vi "Main_Receiver_Localtest.vi"(7 "Tx IQ Sampling\nRate [s/sec]":dbl, 8 "Bitstream Queue Name":string, 9 "Packet Parameters in":T2={"Length of sync sequence (50)"=50, "Number of message bits"=128, "Number of guardbits"=40, "Sync PN sequence order (31)"=31, "Number of header bits"=16, "Packet Pad [samples]"=0}, 10 "QPSK System Parameters":T4={"Samples per Symbol"=8, "symbol map"=[], "Differential PSK"=enum."disable", "PSK type"=0, "M-PSK"=4} {"PSK type" items=["normal", "shifted", "offset"]; "symbol map" format="%.3f"}, 11 "Waveform Queue Name":string) -> ()   [LabVIEW 2014]
uses:
  <instrlib>/niUSRP/niUSRP Fetch Rx Data (CDB Cluster).vi
  <vilib>/addons/Modulation/Digital/General/MT Format Eye Diagram (complex).vi
  <vilib>/addons/Modulation/niDMT.lvlib
panel:
  out "Waveform Graph":dbl[](graph)
  out "Eye Diagram":cluster{"t0":dbl, "dt":dbl, "Y":dbl[]}[](graph)
  out "Sync start":dbl
  out "Max Xcorr Value":dbl
  in  "output cluster":T1
  out "Frames decoded":i32
  out "Max Xcorr Index":i32
  in  "stop":bool
  out "error out":errorcluster
  in  "error in (no error)":errorcluster
  in  "filter parameters":T3={"Alpha"=0.5, "Filter Length"=6, "TX Filter"=enum."Root Raised Cos"} {"Alpha" format="%.2f"}
  in  "USRP IP Address 2":refnum<k15>="192.168.10.1"
  out "Actual Rx Parameters  2":T5={"Rx IQ Sampling\nRate [s/sec]"=200000.0, "Rx\nFrequency [Hz]"=915000000.0, "Rx Gain [dB]"=20.0, "Rx Antenna"="RX1"} {"Rx Gain [dB]" format="%#.6p"; "Rx\nFrequency [Hz]" format="%#.6p"; "Rx IQ Sampling\nRate [s/sec]" format="%#.6p"}
  in  "Rx Parameters 2":T5={"Rx IQ Sampling\nRate [s/sec]"=400000.0, "Rx\nFrequency [Hz]"=5795000000.0, "Rx Gain [dB]"=20.0, "Rx Antenna"="RX1"} {"Rx Gain [dB]" format="%#.6p"; "Rx\nFrequency [Hz]" format="%#.6p"; "Rx IQ Sampling\nRate [s/sec]" format="%#.6p"}
  in  "Acquisition Duration [sec] 2":dbl=0.04 format="%#.6p"
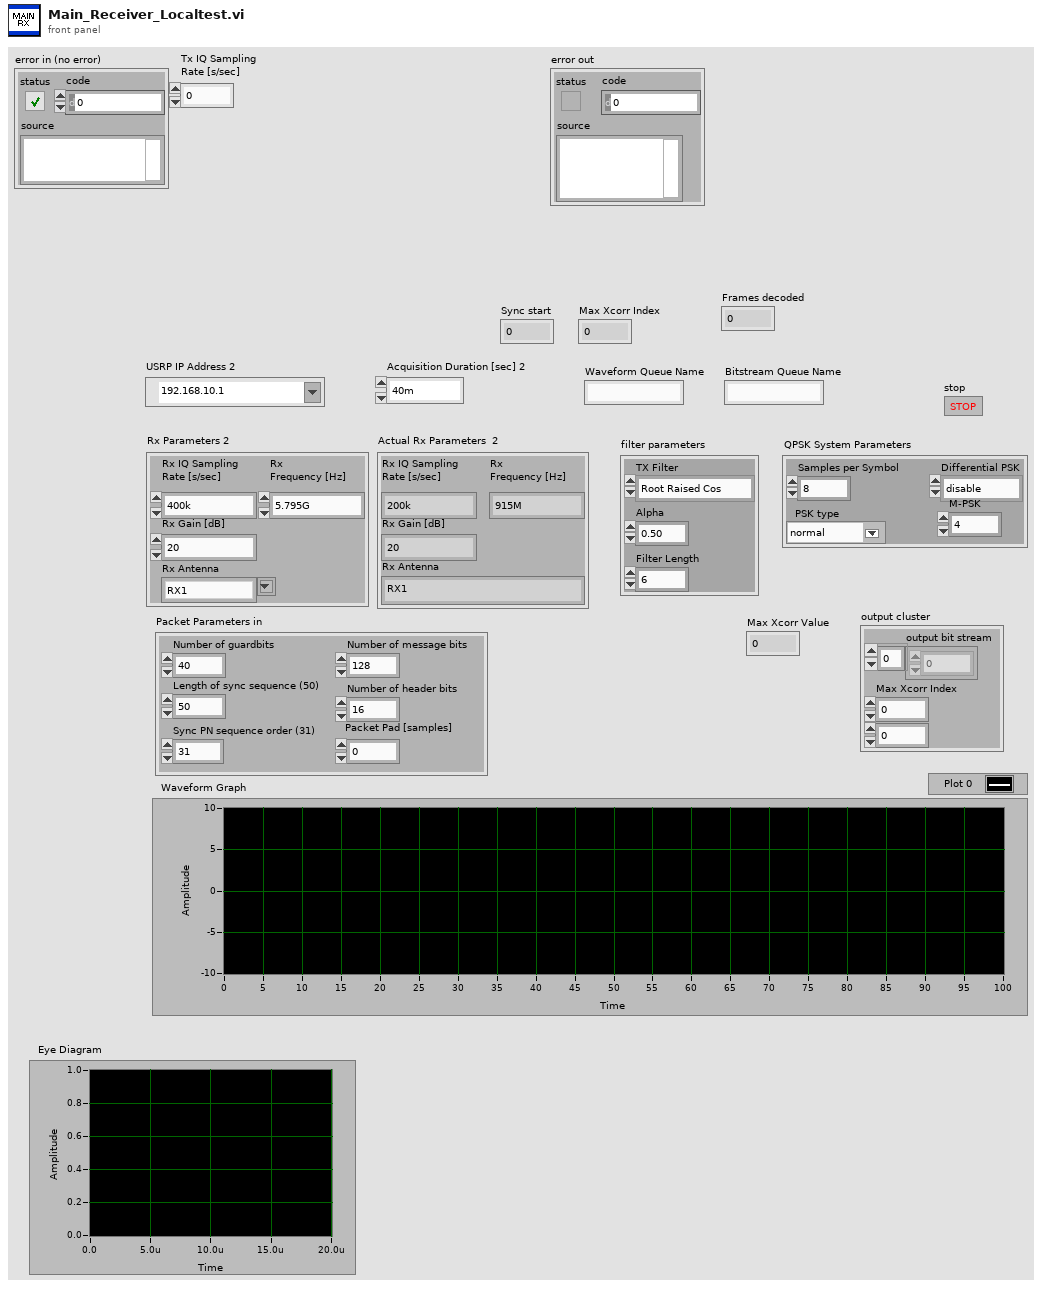
[diagram p1: front panel]
types:
  T1 = cluster{"output bit stream":i8[], "Max Xcorr Index":i32, i32}
  T2 = cluster{"Length of sync sequence (50)":i32, "Number of message bits":i32, "Number of guardbits":i32, "Sync PN sequence order (31)":i32, "Number of header bits":i32, "Packet Pad [samples]":i32}
  T3 = cluster{"Alpha":dbl, "Filter Length":i32, "TX Filter":enum16{"none", "Raised Cosine", "Root Raised Cos", "Gaussian"}}
  T4 = cluster{"Samples per Symbol":i32, "symbol map":cdb[], "Differential PSK":enum16{"disable", "enable"}, "PSK type":u16, "M-PSK":i32}
  T5 = cluster{"Rx IQ Sampling\nRate [s/sec]":dbl, "Rx\nFrequency [Hz]":dbl, "Rx Gain [dB]":dbl, "Rx Antenna":string}
  T6 = cluster{"samples per symbol (16)":i32, "symbol map":cdb[], "differential PSK":enum16{"disable", "enable"}, "PSK type":u16}
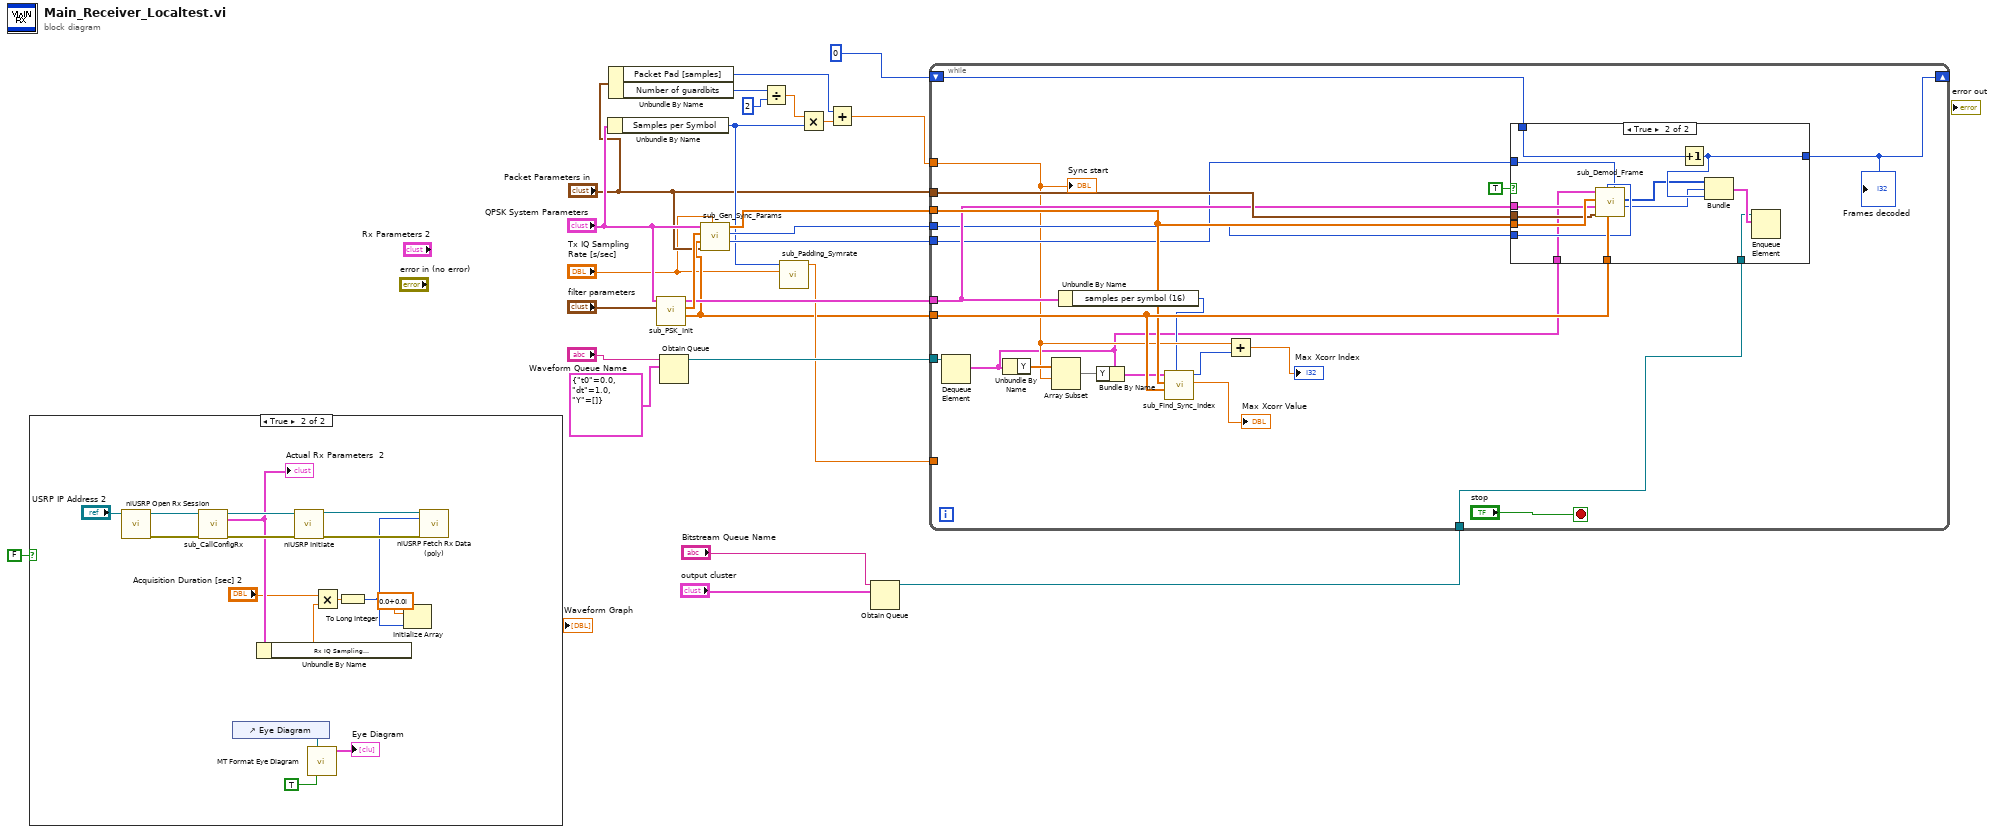
[diagram p0: block diagram]
diagram:
  n1 = case shown="True" FALSE {
    frame False {
    }
    frame True {
      n2 = call <instrlib>:"niUSRP Open Rx Session.vi"("device names"="USRP IP Address 2") -> ("session handle out"=w39:refnum<k15>, "error out"=w40:errorcluster)  [unwired: 13 in]
      n3 = call "sub_CallConfigRx.vi"("session handle"=w39, "error in"=w40) -> ("session handle out"=w38:refnum<k15>, "Actual Rx Parameters"=w35:T5, "error out"=w37:errorcluster)  [unwired: 11 in]
      "Actual Rx Parameters  2" <- w35
      n4 = control-ref of="Eye Diagram"() -> (w28:refnum<vi>)
      n5 = Unbundle By Name(w35) -> ("Rx IQ Sampling\nRate [s/sec]"=w33:dbl)
      n6 = call <instrlib>:"niUSRP Initiate.vi"("session handle"=w38, "error in (no error)"=w37) -> ("session handle out"=w32:refnum<k15>, "error out"=w31:errorcluster)  [unwired: 12 in]
      n7 = call-poly <vilib>:"MT Format Eye Diagram.vi"("eye diagram reference"=w28, "autoscale"=TRUE) -> ("eye diagram"=→"Eye Diagram":cluster{"t0":dbl, "dt":dbl, "Y":dbl[]}[])  [unwired: 5 in, 8 out]
      n8 = Multiply(x="Acquisition Duration [sec] 2", y=w33) -> (x*y=w42:dbl)
      n9 = To Long Integer(number=w42) -> (32bit integer=w30:i32)
      n10 = Initialize Array(cdb 0.0+0.0i ("element"), w30) -> ()  [unwired: 1 out]
      n11 = call-poly <instrlib>:"niUSRP Fetch Rx Data (poly).vi"("session handle"=w32, "number of samples"=w30, "error in (no error)"=w31) -> ()  [unwired: 9 in, 4 out]
    }
  }
  n12 = Unbundle By Name("QPSK System Parameters") -> ("Samples per Symbol"=w7:i32)
  n13 = Unbundle By Name("Packet Parameters in") -> ("Packet Pad [samples]"=w5:i32, "Number of guardbits"=w9:i32)
  n14 = call "sub_PSK_Init.vi"("filter parameters in"="filter parameters", "QPSK System Parameters in"="QPSK System Parameters") -> ("matched filter coefficients"=w3:dbl[], "pulse shaping filter coefficients"=w25:dbl[], "PSK system parameters"=w23:T6)  [unwired: 7 in]
  n15 = Obtain Queue(name (unnamed)="Waveform Queue Name", element data type=cluster{"t0":dbl, "dt":dbl, "Y":cdb[]} {"t0"=0.0, "dt"=1.0, "Y"=[]} ("s? t:f")) -> (queue out=w20:refnum<queue>)  [unwired: 3 in, 2 out]
  n16 = call "sub_Gen_Sync_Params.vi"("IQ Sampling\nRate [s/sec]"="Tx IQ Sampling\nRate [s/sec]", "Packet Parameters in"="Packet Parameters in", "matched filter coefficients"=w3, "pulse shaping filter coefficients"=w25, "QPSK System Parameters in"="QPSK System Parameters") -> ("Frame Length (samples)"=w11:i32, "Expected Xcorr Index"=w12:i32, "Sync Sequence Waveform"=w15:cdb[])  [unwired: 3 in, 1 out]
  n17 = Divide(x=w9, y=2) -> (x/y=w8:dbl)
  n18 = call "sub_Padding_Symrate.vi"("Tx IQ Sampling\nRate [s/sec]"="Tx IQ Sampling\nRate [s/sec]", "Samples per Symbol"=w7) -> ("Symbol Rate"=w10:dbl)  [unwired: 8 in, 1 out]
  n19 = Multiply(x=w8, y=w7) -> (x*y=w6:dbl)
  n20 = Add(x=w5, y=w6) -> (x+y=w4:dbl)
  n21 = Obtain Queue(name (unnamed)="Bitstream Queue Name", element data type="output cluster") -> (queue out=w19:refnum<queue>)  [unwired: 3 in, 2 out]
  n22 = while {
    tunnel: w3 -> [w63]
    tunnel: w12 -> [w57]
    tunnel: w15 -> [w62]
    tunnel: "Packet Parameters in" -> [w61]
    tunnel: w23 -> [w60]
    tunnel: w11 -> [w56]
    tunnel: w20 -> [w59]
    tunnel: w19 -> [w55]
    shift-right: [w53] -> _
    shift-left: 0 ("index") -> [w54]
    tunnel: w4 -> [w45]
    tunnel: w10 -> [_]
    stop <- "stop" stop-if-true
    n23 = Dequeue Element(queue=w59) -> (element=w43:cluster{"t0":dbl, "dt":dbl, "Y":cdb[]})  [unwired: 2 in, 3 out]
    n24 = Unbundle By Name(w43) -> ("Y"=w52:cdb[])
    n25 = Array Subset(array=w52, index=w45) -> (w51:cdb[])  [unwired: 1 in]
    n26 = Unbundle By Name(w60) -> ("samples per symbol (16)"=w44:i32)
    n27 = Bundle By Name(cluster=w43, "Y"=w51) -> (w50:cluster{"t0":dbl, "dt":dbl, "Y":cdb[]})
    n28 = call "sub_Find_Sync_Index.vi"("samples per symbol (16)"=w44, "matched filter coefficients"=w63, "Sync Sequence Waveform"=w62, "Input Complex Waveform"=w50) -> ("Max Xcorr Value"=→"Max Xcorr Value":dbl, "Max Xcorr Index"=w46:i32)  [unwired: 5 in, 1 out]
    n29 = Add(x=w45, y=w46) -> (x+y=→"Max Xcorr Index":dbl)
    n30 = case shown="True" TRUE {
      tunnel: w62 -> [_ w77]
      tunnel: w60 -> [_ w76]
      tunnel: w61 -> [_ w75]
      tunnel: w63 -> [_ w74]
      tunnel: w57 -> [_ w73]
      tunnel: w56 -> [_ w72]
      tunnel: w55 -> [_ w70]
      tunnel: [w64 w68] -> w53
      tunnel: w54 -> [w64 w69]
      tunnel: w43 -> [_ w65]
      frame False {
      }
      frame True {
        n31 = call "sub_Demod_Frame.vi"("Packet Length [samples]"=w72, "matched filter coefficients"=w74, "Expected Xcorr Index"=w73, "Packet Parameters in"=w75, "PSK system parameters"=w76, "Sync Sequence Waveform"=w77, "Input Complex Waveform"=w65) -> ("Max Xcorr Index"=w66:i32, "output bit stream"=w67:i8[])  [unwired: 2 in, 1 out]
        n32 = Increment(x=w69) -> (x+1=w68:i32)
        n33 = Bundle("output bit stream"=w67, "Max Xcorr Index"=w66, w68) -> (w71:T1)  [unwired: 1 in]
        n34 = Enqueue Element(queue=w70, element=w71) -> ()  [unwired: 2 in, 3 out]
      }
    }
    "Frames decoded" <- w53
    "Sync start" <- w45
  }
